vi "SubI16.vi"(4 "y":i16, 5 "x":i16) -> (1 "x-y":i16, 2 "Overflow?":bool)   [LabVIEW 2017, in "GPOverflow.lvlib"]
doc: "Subtracts <B>y</B> from <B>x</B> keeping track of numeric overflow.\n\n<B>Overflow?</B> will be True if positive or negative overflow occurred. The output will saturate in case of overflow.\n\nThis VI is inlined.\n\nSteen Schmidt\nGPower\n8/8 2013"
uses:
  GPOverflow.lvlib
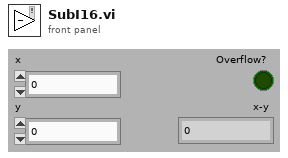
[diagram p1: front panel]
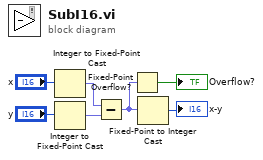
[diagram p0: block diagram]
diagram:
  n1 = Integer to Fixed-Point Cast(integer="x") -> (fixed-point=w5:fxp<+/-,16,16>)  [unwired: 1 in]
  n2 = Integer to Fixed-Point Cast(integer="y") -> (fixed-point=w4:fxp<+/-,16,16>)  [unwired: 1 in]
  n3 = Subtract(x=w5, y=w4) -> (x-y=w3:fxp<+/-,16,16>)
  n4 = Fixed-Point Overflow?(1:w3) -> (0:→"Overflow?":bool)
  n5 = Fixed-Point to Integer Cast(1:w3) -> (0:→"x-y":i16)
